vi "resetDAQ.vi"(8 "error in (no error)":errorcluster, 11 "Instrument.Lockin in":refnum<class "Instrument.Lockin.lvclass">) -> (0 "error out":errorcluster, 3 "Instrument.Lockin out":refnum<class "Instrument.Lockin.lvclass">)   [LabVIEW 2019, in "Instrument.Lockin.lvclass"]
doc: "API to put lockin into remote mode.\n\nIf address=\"\", this API reads from localhost\nIf address is remote lockin, you need to add this computer to allowed whitelist on the lockin computer you are trying to access."
uses:
  Instrument.Lockin.lvclass
  Instrument.DAQ/Typedefs/Set State-enum.ctl
  Instrument.DAQ/Instrument.DAQ.lvclass
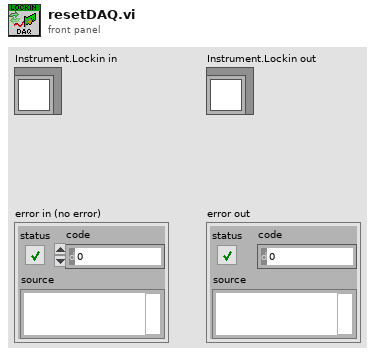
[diagram p1: front panel]
types:
  T1 = typedef "Instrument.DAQ.lvclass/Set State-enum.ctl" = enum16{"start", "stop", "reset", "start sweep", "stop sweep"}
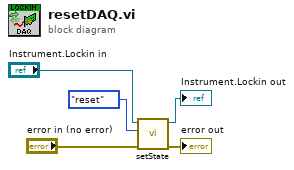
[diagram p0: block diagram]
diagram:
  n1 = call "setState.vi"("error in (no error)"="error in (no error)", "State"=Set_State-enum."reset" ("Data out"), "Instrument.Lockin in"="Instrument.Lockin in") -> ("error out"=→"error out":errorcluster, "Instrument.Lockin out"=→"Instrument.Lockin out":refnum<class "Instrument.Lockin.lvclass">)  [unwired: 7 in]
